vi "Launch New Station.vi"(8 "error in":errorcluster, 11 "OPC Server in":refnum<class "OPC Server.lvclass">) -> (0 "error out":errorcluster, 3 "OPC Server out":refnum<class "OPC Server.lvclass">)   [LabVIEW 2021, in "OPC Server.lvlib" / "OPC Server.lvclass"]
uses:
  OPC Server.lvclass
  C:/Program Files/National Instruments/LabVIEW 2021/vi.lib/ActorFramework/Actor/Actor.lvclass
  Station Panel/Station Panel Actor/Panel.lvclass
  <vilib>/OPCUA/controls/OPC UA Server Refnum.ctl
  OPC Server.lvclass/OPC Server.ctl
  Station/Station Messages/Set Node IDs Msg/Set Node IDs Msg.lvclass/Set Node IDs Msg.ctl
  <vilib>/ActorFramework/Message Enqueuer/Message Enqueuer.lvclass/Message Enqueuer.ctl
  Station/Station Messages/Set Window Title Msg/Set Window Title Msg.lvclass/Set Window Title Msg.ctl
  Station Panel/Panel Messages/Pause Resume OPC UA Msg/Pause Resume OPC UA Msg.lvclass/Pause Resume OPC UA Msg.ctl
  <vilib>/ActorFramework/Message Enqueuer/Enqueue.vi
  Station/Station Messages/Set Node IDs Msg/Set Node IDs Msg.lvclass
  C:/Program Files/National Instruments/LabVIEW 2021/vi.lib/ActorFramework/Message/Message.lvclass
  Station/Station Messages/Set Window Title Msg/Set Window Title Msg.lvclass
  Station Panel/Panel Messages/Pause Resume OPC UA Msg/Pause Resume OPC UA Msg.lvclass
  <vilib>/ActorFramework/Message Priority Queue/Priority Enqueue.vi
  <vilib>/ActorFramework/Actor/Actor.lvclass
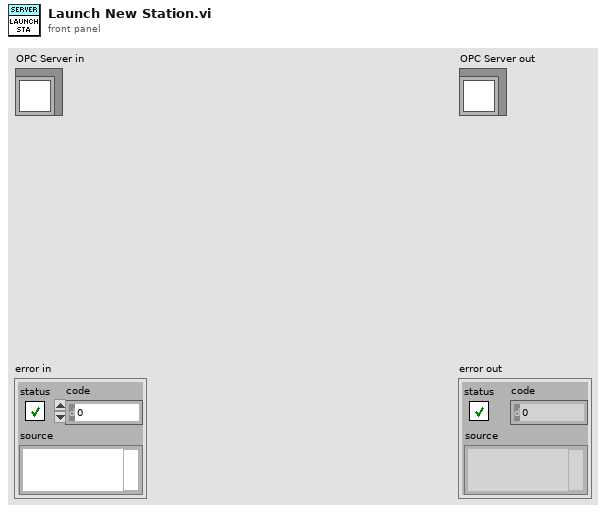
[diagram p1: front panel]
types:
  T1 = typedef "OPC UA Server Refnum.ctl" = refnum<k21>
  T2 = cluster{"Rx Folder Node ID":string, "Tx Folder Node ID":string, "OPC UA server refnum":T1}
  T3 = map{string, refnum<class "Message Enqueuer.lvclass">}
  T4 = typedef "NodeId.ctl" = string
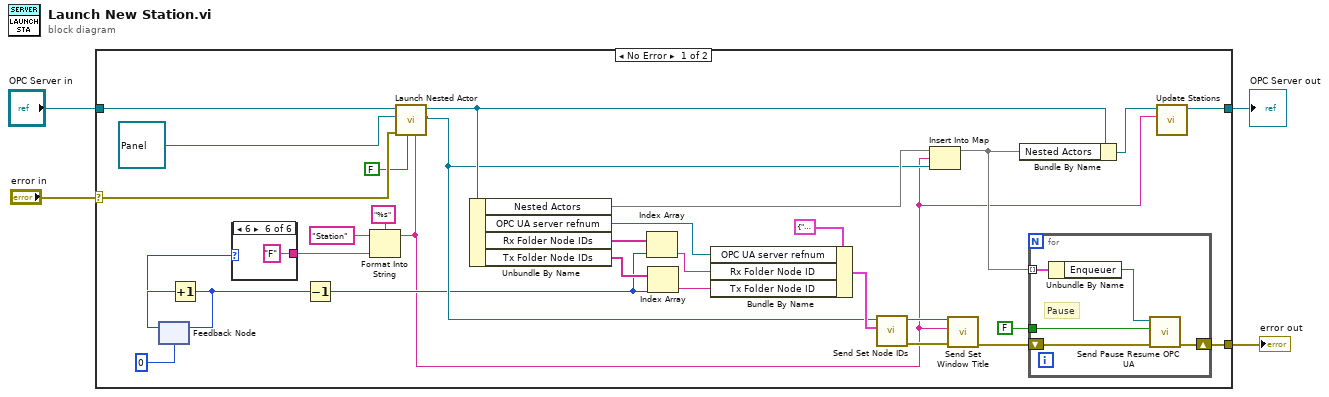
[diagram p0: block diagram]
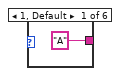
[diagram p2: hidden frame]
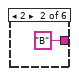
[diagram p3: hidden frame]
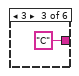
[diagram p4: hidden frame]
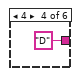
[diagram p5: hidden frame]
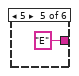
[diagram p6: hidden frame]
diagram:
  n1 = case shown="No Error" "error in" {
    selector: "error in" -> [w33 w47]
    tunnel: [w11 w47] -> w3
    tunnel: [w26 w46] -> w1
    tunnel: "OPC Server in" -> [w34 w46]
    frame No Error {
      n2 = feedback #1(0) -> (w31:i32)
      n3 = Increment(x=w31) -> (x+1=w7:i32)
      n4 = feedback-in #1(w7) -> ()
      n5 = case shown="6" w7 {
        tunnel: ["A" "B" "C" "D" "E" "F"] -> w9
        frame 1, Default {
        }
        frame 2 {
        }
        frame 3 {
        }
        frame 4 {
        }
        frame 5 {
        }
        frame 6 {
        }
      }
      n6 = Decrement(x=w7) -> (x-1=w6:i32)
      n7 = Format Into String(format string="%s", initial string="Station", w9) -> (resulting string=w5:string)  [unwired: 1 in, 1 out]
      n8 = call <vilib>:"Launch Nested Actor.vi"("Debug Alias"=w5, "Open Actor Core front panel? (F)"=FALSE, "error in (no error)"=w33, "Nested Actor"=refnum<class "Panel.lvclass"> refnum ("Panel.lvlib:Panel.lvclass"), "Caller Actor in"=w34) -> ("Nested Actor's Enqueuer"=w14:refnum<class "Message Enqueuer.lvclass">, "Caller Actor out"=w27:refnum<class "OPC Server.lvclass">)  [unwired: 4 in, 1 out]
      n9 = Unbundle By Name(w27) -> ("Nested Actors"=w28:T3, "OPC UA server refnum"=w18:T1, "Rx Folder Node IDs"=w24:T4[], "Tx Folder Node IDs"=w23:T4[])
      n10 = Index Array(array=w24, index=w6) -> (element=w17:T4)
      n11 = Index Array(array=w23, index=w6) -> (element=w20:T4)
      n12 = Bundle By Name(cluster=T2 {"Rx Folder Node ID"="", "Tx Folder Node ID"="", "OPC UA server refnum"=""} ("FolderIDs"), "OPC UA server refnum"=w18, "Rx Folder Node ID"=w17, "Tx Folder Node ID"=w20) -> (w16:T2)
      n13 = call "Send Set Node IDs.vi"("FolderIDs"=w16, "Message Enqueuer"=w14) -> ("error out"=w22:errorcluster, "Message Enqueuer out"=w21:refnum<class "Message Enqueuer.lvclass">)  [unwired: 8 in]
      n14 = Insert Into Map(map in=w28, key=w5, value=w14) -> (map out=w10:T3)  [unwired: 2 out]
      n15 = call "Send Set Window Title.vi"("error in (no error)"=w22, "FP Window:Title"=w5, "Message Enqueuer"=w21) -> ("error out"=w12:errorcluster)  [unwired: 7 in, 1 out]
      n16 = Bundle By Name(cluster=w27, "Nested Actors"=w10) -> (w25:refnum<class "OPC Server.lvclass">)
      n17 = for {
        tunnel: FALSE ("Pause/Resume") -> [w45]
        shift-right: [w43] -> w11
        shift-left: w12 -> [w44]
        tunnel: w10 -> [w42] mode=indexing
        # "Pause"
        n18 = Unbundle By Name(w42) -> ("Enqueuer"=w41:refnum<class "Message Enqueuer.lvclass">)
        n19 = call "Send Pause Resume OPC UA.vi"("error in (no error)"=w44, "Pause/Resume"=w45, "Message Enqueuer"=w41) -> ("error out"=w43:errorcluster)  [unwired: 7 in, 1 out]
      }
      n20 = call "Update Stations.vi"("Combo Value"=w5, "OPC Server in"=w25) -> ("OPC Server out"=w26:refnum<class "OPC Server.lvclass">)  [unwired: 8 in, 1 out]
    }
    frame Error {
    }
  }
  "error out" <- w3
  "OPC Server out" <- w1
